vi "Ref to LVClass.vi"(8 "error in (no error)":errorcluster, 11 "ProjectItem in":refnum<vi>) -> (0 "error out":errorcluster, 3 "LVClassLibrary out":refnum<vi>)   [LabVIEW 2019, in "gRPC Scripting Tools.lvlib"]
uses:
  gRPC Scripting Tools.lvlib
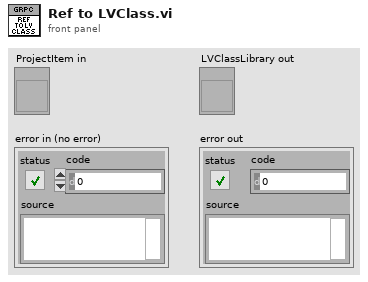
[diagram p1: front panel]
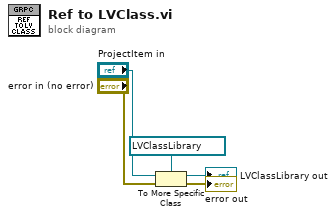
[diagram p0: block diagram]
diagram:
  n1 = To More Specific Class(target class=refnum<vi> refnum ("LVClassLibrary out"), reference="ProjectItem in", error in="error in (no error)") -> (specific class reference=→"LVClassLibrary out":refnum<vi>, error out=→"error out":errorcluster)
